vi "Fingerprint.vi"(7 "Address":string, 8 "Error In":errorcluster) -> (0 "Error Out":errorcluster)   [LabVIEW 2018, in "Tests.lvlib" / "Session.lvlib"]
uses:
  Session.lvlib
  src/Toolkit/Session/Type Definitions/Host Key Hash Types.ctl
  <vilib>/addons/_JKI Toolkits/Caraya/classes/Test/Test.lvclass
  src/Toolkit/SSH/SSH.lvclass
  src/Toolkit/Session/Session.lvclass
  <vilib>/addons/_JKI Toolkits/Caraya/classes/Assert/Assert.lvclass
  Tests.lvlib
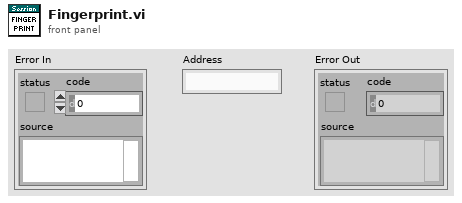
[diagram p1: front panel]
types:
  T1 = typedef "Toolkit.lvlib/Session.lvclass/Host Key Hash Types.ctl" = i32
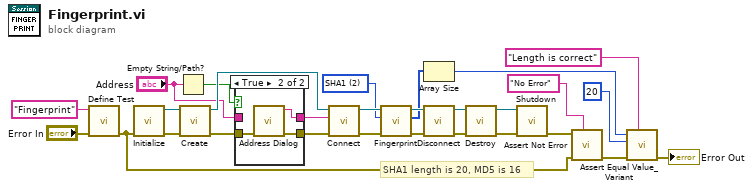
[diagram p0: block diagram]
diagram:
  w1 = T1 2 items=["MD5"=1, "SHA1"=2] ("Type")
  # "SHA1 length is 20, MD5 is 16"
  n1 = call <vilib>:"Define Test.vi"("error in (no error)"="Error In", "Label (VI Title)"="Fingerprint") -> ("error out"=w20:errorcluster)  [unwired: 9 in]
  n2 = call "Initialize.vi"("Error In"=w20) -> ("Error Out"=w26:errorcluster, "SSH"=w25:refnum<class "SSH.lvclass">)  [unwired: 9 in]
  n3 = Empty String/Path?(string/path="Address") -> (empty?=w6:bool)
  n4 = call "Create.vi"("Error In"=w26, "SSH"=w25) -> ("Error Out"=w3:errorcluster, "Sesssion"=w18:refnum<class "Session.lvclass">)  [unwired: 8 in]
  n5 = case shown="True" w6 {
    tunnel: w3 -> [w29 w33]
    tunnel: [w29 w32] -> w2
    tunnel: [w30 w31] -> w5
    tunnel: "Address" -> [w30 _]
    frame False {
    }
    frame True {
      n6 = call "Address Dialog.vi"("Error In"=w33) -> ("Error Out"=w32:errorcluster, "Address Out"=w31:string)  [unwired: 9 in]
    }
  }
  n7 = call "Connect.vi"("Error In"=w2, "Address"=w5, "Session In"=w18) -> ("Error Out"=w14:errorcluster, "Sesssion Out"=w15:refnum<class "Session.lvclass">)  [unwired: 7 in]
  n8 = call "Fingerprint.vi"("Error In"=w14, "Type"=w1, "Session In"=w15) -> ("Error Out"=w12:errorcluster, "Fingerprint"=w10:u8[], "Sesssion Out"=w13:refnum<class "Session.lvclass">)  [unwired: 6 in]
  n9 = Array Size(array=w10) -> (size(s)=w9:i32)
  n10 = call "Disconnect.vi"("Error In"=w12, "Session In"=w13) -> ("Error Out"=w16:errorcluster, "Sesssion Out"=w17:refnum<class "Session.lvclass">)  [unwired: 8 in]
  n11 = call "Destroy.vi"("Error In"=w16, "Session"=w17) -> ("Error Out"=w23:errorcluster, "SSH"=w24:refnum<class "SSH.lvclass">)  [unwired: 8 in]
  n12 = call "Shutdown.vi"("Error In"=w23, "SSH"=w24) -> ("Error Out"=w22:errorcluster)  [unwired: 9 in]
  n13 = call <vilib>:"Assert Not Error.vi"("Label"="No Error", "error in (no error)"=w20, "Not Error?"=w22) -> ("error out"=w19:errorcluster)  [unwired: 8 in]
  n14 = call <vilib>:"Assert Equal Value_Variant.vi"("Label"="Length is correct", "error in (no error)"=w19, "Y"=20 ("size(s)"), "X"=w9) -> ("error out"=→"Error Out":errorcluster)  [unwired: 7 in]
